vi "Control Experiment.setUIconfig.vi"(8 "error in (no error)":errorcluster, 10 "UI Configuration":T1={"Metadata"={"Sample (SAXXXX)"="TEST", "Device (YYYYMMDD)"="20200113", "Description"="this is a test", "Username"="Patrick", "Default Path"=path "C:/DataTemp"}, "Number of AI"=8, "UI Channels []"=[], "Instruments"={"Lockin Address"="", "Krohn Hite?"=FALSE, "KH Addresses"=[], "Strain Cell?"=TRUE, "Strain Cell Address"="", "C Bridge?"=TRUE, "Capacitance Bridge Address"="", "Instrument"=enum."----- AFM/EBL -----"}, "Krohn Hite"={"Defualt Shunt Resistor"=enum."50k Ohms", "Default Gain"=enum."10x", "Coupling"=enum."DC", "Bandwidth Filter"=enum."ON"}} {"UI Channels []"."KH"."Channel" items=["A 1"]}, 11 "Control Experiment":refnum<class "SMO.Control Experiment.lvclass">) -> (0 "error out":errorcluster, 3 "Control Experiment out":refnum<class "SMO.Control Experiment.lvclass">)   [LabVIEW 2019, in "SMO.Control Experiment.lvclass"]
doc: "---------------------------------------------------------------\nJKI State Machine Objects™\nhttp://jki.net/state-machine-objects/\nCopyright (C) 2005-2015, JKI <info@jki.net>\nALL RIGHTS RESERVEDJKI State Machine Objects (SMO) 1.0.0.4\nJKI - JKI\nCopyright (c) 2015, JKI"
uses:
  SMO.Control Experiment.lvclass
  SMO.Control Experiment UI/Typedefs/UI Config--Cluster.ctl
  SMO.Control Experiment UI/Typedefs/UI Channels--Cluster.ctl
  SMO.Control Experiment UI/Typedefs/UI Channels.AI--Cluster.ctl
  SMO.Control Experiment UI/Typedefs/UI Channels.Device--Cluster.ctl
  Private/Control Experiment SM/Typedefs/KH Mode-enum.ctl
  SMO.Control Experiment UI/Typedefs/UI Channels.KH--Cluster.ctl
  <userlib>/LevyLab/Krohn Hite 7008/typedefs/Input Configuration-Enum.ctl
  <userlib>/LevyLab/Krohn Hite 7008/typedefs/Gain-Enum.ctl
  <userlib>/LevyLab/Krohn Hite 7008/typedefs/Shunt-Enum.ctl
  SMO.Control Experiment UI/Typedefs/UI Channels.AO--Cluster.ctl
  Private/Control Experiment SM/Typedefs/Instrument--enum.ctl
  <userlib>/LevyLab/Krohn Hite 7008/typedefs/Coupling-Enum.ctl
  <userlib>/LevyLab/Krohn Hite 7008/typedefs/Filter-Enum.ctl
  SMO.Control Experiment.lvclass/SMO.Control Experiment.ctl
  SMO.Control Experiment UI/SMO.Control Experiment UI.lvclass
  <userlib>/LevyLab/Krohn Hite 7008/Instrument.KH7008.lvclass
panel:
  # "For instructions on how to use the JKI State Machine Objects, examples and video tutorials, visit:\nhttp://jki.net/state-machine-objects/\n\nJKI State Machine Objects™\nhttp://jki.net/state-machine-objects/\nCopyright (C) 2005-2015, JKI <info@jki.net>\nALL RIGHTS RESERVED"
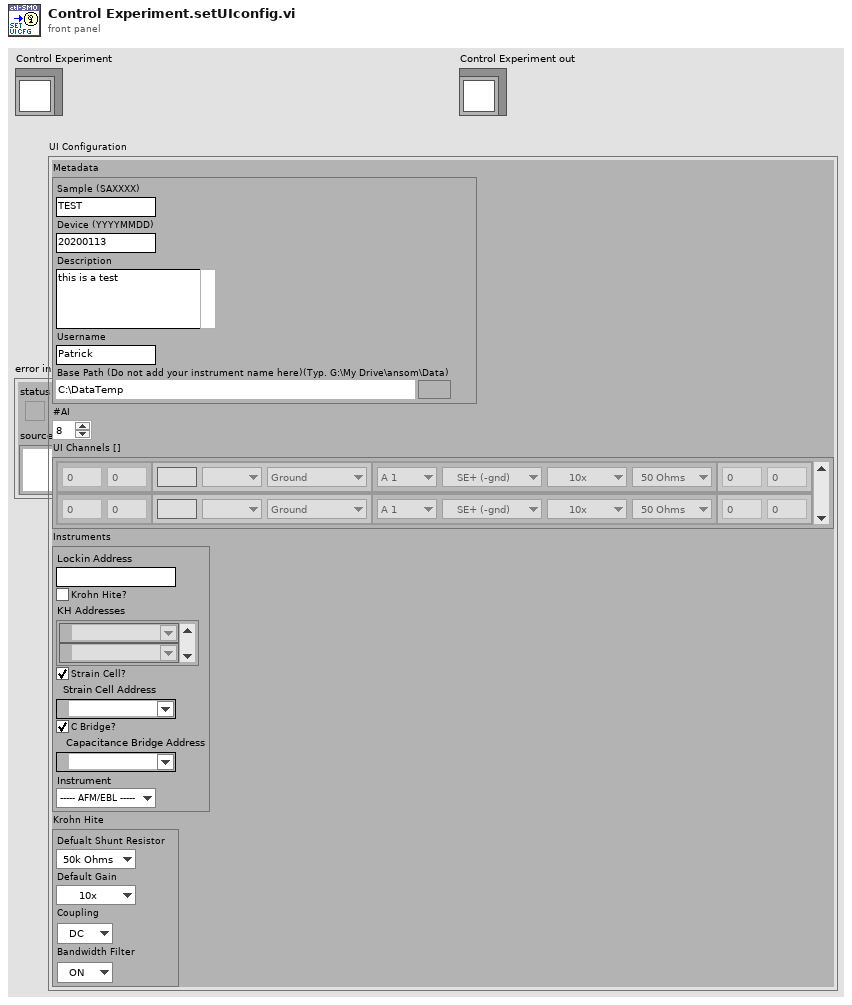
[diagram p1: front panel]
types:
  T1 = typedef "SMO.Control Experiment.lvclass/UI Config--Cluster.ctl" = cluster{"Metadata":cluster{"Sample (SAXXXX)":string, "Device (YYYYMMDD)":string, "Description":string, "Username":string, "Default Path":path}, "Number of AI":i32, "UI Channels []":T2[], "Instruments":cluster{"Lockin Address":string, "Krohn Hite?":bool, "KH Addresses":refnum<visa-resource-name>[], "Strain Cell?":bool, "Strain Cell Address":refnum<visa-resource-name>, "C Bridge?":bool, "Capacitance Bridge Address":refnum<visa-resource-name>, "Instrument":T11}, "Krohn Hite":cluster{"Defualt Shunt Resistor":T9, "Default Gain":T8, "Coupling":T12, "Bandwidth Filter":T13}}
  T2 = typedef "SMO.Control Experiment UI.lvclass/UI Channels--Cluster.ctl" = cluster{"AI":T3, "Device":T4, "KH":T6, "AO":T10}
  T3 = typedef "SMO.Control Experiment UI.lvclass/UI Channels.AI--Cluster.ctl" = cluster{"Channel":u32, "Gain":dbl}
  T4 = typedef "SMO.Control Experiment UI.lvclass/UI Channels.Device--Cluster.ctl" = cluster{"Electrode":string, "Configuration":T5, "Label":u16}
  T5 = typedef "SMO.Control Experiment.lvclass/KH Mode-enum.ctl" = enum16{"Ground", "Current", "Voltage (SE)", "Voltage (Diff)", "Gate"}
  T6 = typedef "SMO.Control Experiment UI.lvclass/UI Channels.KH--Cluster.ctl" = cluster{"Channel":u16, "Configuration":T7, "Gain":T8, "Shunt Resistor":T9}
  T7 = typedef "Instrument.KH7008.lvclass/Input Configuration-Enum.ctl" = enum16{"Ground", "SE+ (-gnd)", "SE- (+gnd)", "Differential"}
  T8 = typedef "Instrument.KH7008.lvclass/Gain-Enum.ctl" = enum16{"1x", "10x", "100x", "1000x"}
  T9 = typedef "Instrument.KH7008.lvclass/Shunt-Enum.ctl" = enum16{"Open", "50 Ohms", "500 Ohms", "5k Ohms", "50k Ohms", "10M Ohm"}
  T10 = typedef "SMO.Control Experiment UI.lvclass/UI Channels.AO--Cluster.ctl" = cluster{"Channel":u32, "Gain":dbl}
  T11 = typedef "SMO.Control Experiment.lvclass/Instrument--enum.ctl" = enum16{"----- AFM/EBL -----", "AGILENT", "CYPHER", "Gemini2", "JEOL", "MFP3D", "----- Cryostat -----", "CF900", "DR200", "MNK", "PPMS 1", "PPMS 2", "PPMS 3", "----- Optics -----", "THz 1", "THz 2"}
  T12 = typedef "Instrument.KH7008.lvclass/Coupling-Enum.ctl" = enum16{"AC", "DC"}
  T13 = typedef "Instrument.KH7008.lvclass/Filter-Enum.ctl" = enum16{"OFF", "ON"}
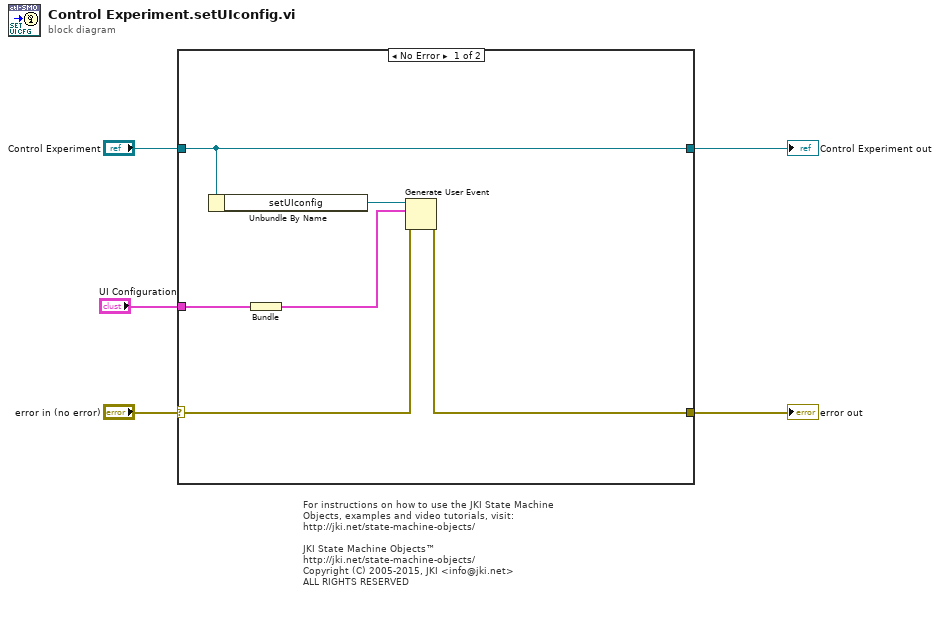
[diagram p0: block diagram]
diagram:
  # "For instructions on how to use the JKI State Machine Objects, examples and video tutorials, visit:\nhttp://jki.net/state-machine-objects/\n\nJKI State Machine Objects™\nhttp://jki.net/state-machine-objects/\nCopyright (C) 2005-2015, JKI <info@jki.net>\nALL RIGHTS RESERVED"
  n1 = case shown="No Error" "error in (no error)" {
    selector: "error in (no error)" -> [w11 w13]
    tunnel: [w9 w13] -> w4
    tunnel: [w8 w12] -> w5
    tunnel: "Control Experiment" -> [w8 w12]
    tunnel: "UI Configuration" -> [w7 _]
    frame No Error {
      n2 = Unbundle By Name(w8) -> ("setUIconfig"=w10:refnum<user-event>)
      n3 = Bundle("UI Configuration"=w7) -> (w6:cluster{"UI Configuration":T1})  [unwired: 1 in]
      n4 = Generate User Event(user event=w10, event data cluster=w6, error in=w11) -> (error out=w9:errorcluster)  [unwired: 1 in, 1 out]
    }
    frame Error {
    }
  }
  "error out" <- w4
  "Control Experiment out" <- w5
